vi "Rebundle.vi"() -> ()   [LabVIEW 2010]
uses:
  Cluster Typedef.ctl
panel:
  out "output cluster":T1={"Enum"=enum."Option 1", "Variant"=variant}
  in  "input cluster":T1={"Enum"=enum."Option 1", "Variant"=variant}
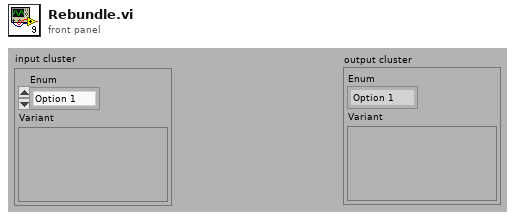
[diagram p1: front panel]
types:
  T1 = typedef "Cluster Typedef.ctl" = cluster{"Enum":enum16{"Option 0", "Option 1"}, "Variant":variant}
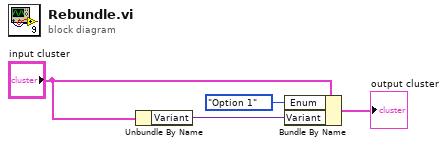
[diagram p0: block diagram]
diagram:
  n1 = Unbundle By Name("input cluster") -> ("Variant"=w4:variant)
  n2 = Bundle By Name(cluster="input cluster", "Enum"=enum16{"Option 0", "Option 1"}."Option 1", "Variant"=w4) -> (→"output cluster":T1)
